vi "P116x2ch_WriteAuto.vi"(5 "P116x2":T1, 7 "Enable(T)":bool=TRUE, 8 "error in (no error)":errorcluster, 9 "RateSP":T2, 10 "NuevoSP":T2, 11 "VISA Eurotherm":refnum<visa-resource-name>) -> (0 "error out":errorcluster, 1 "RateSP_out":T2, 2 "NuevoSP_out":T2)   [LabVIEW 2017]
uses:
  2xP116.ctl
  _P2024_P116x2w.ctl
  Address.ctl
  Eurotherm_2023_Module.ctl
  P2024 TB ICB GLOBALES.vi
panel:
  out "PV":T2
  out "WorkingSP":T2
  out "TargetSP":T2
  in  "Cancel":bool
  in  "Write":bool
  in  "Delay Time (s)":dbl=0.1
  # "Setpoint auto controladores P116"
  # "C/min"
  # "C"
  # "C"
  # "C"
  # "C"
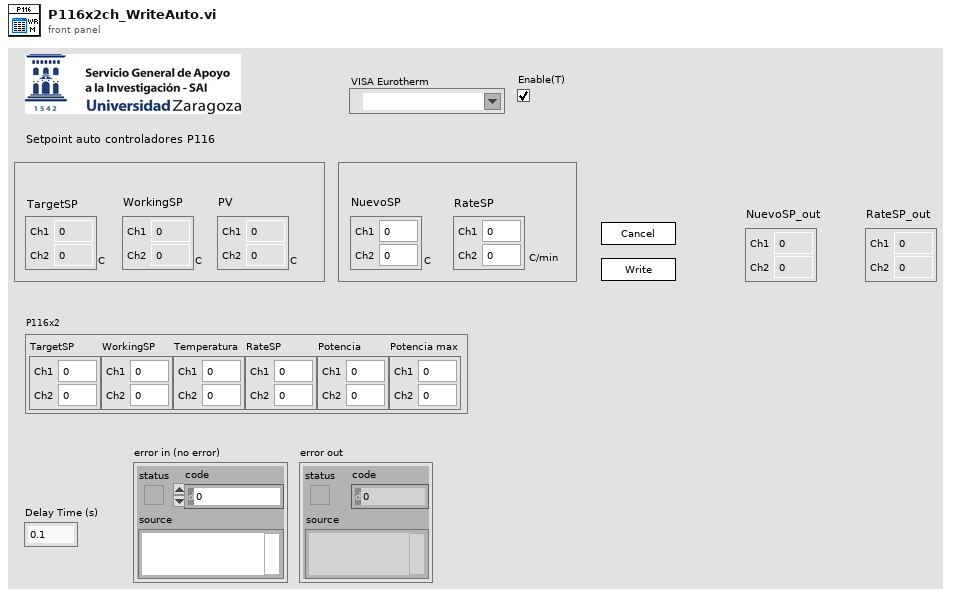
[diagram p1: front panel]
types:
  T1 = typedef "_P2024_P116x2w.ctl" = cluster{"TargetSP":T2, "WorkingSP":T2, "Temperatura":T2, "RateSP":T2, "Potencia":T2, "Potencia max":T2}
  T2 = typedef "2xP116.ctl" = cluster{"Ch1":dbl, "Ch2":dbl}
  T3 = typedef "_P2024 COMMS.ctl" = cluster{"Alicat":refnum<visa-resource-name>, "eAlic":bool, "Eurotherm":refnum<visa-resource-name>, "eEurot":bool, "Balanza":refnum<visa-resource-name>, "eBal":bool, "Valvula":refnum<visa-resource-name>, "eVal":bool}
  T4 = typedef "Eurotherm_2023_Module.ctl" = enum16{"Initialize", "Write setpoint", "Read data", "Write ramp rate", "Set constante proporcional", "Set constante integral", "Set constante diferencial", "Set ouput limit LOW", "Set ouput limit HIGH", "Shutdown"}
  T5 = typedef "Address.ctl" = enum16{"Add 1", "Add 2", "Add 3", "Add 4", "Add 5", "Add 6", "Add 10", "Add 11", "Add 12", "Add 13"}
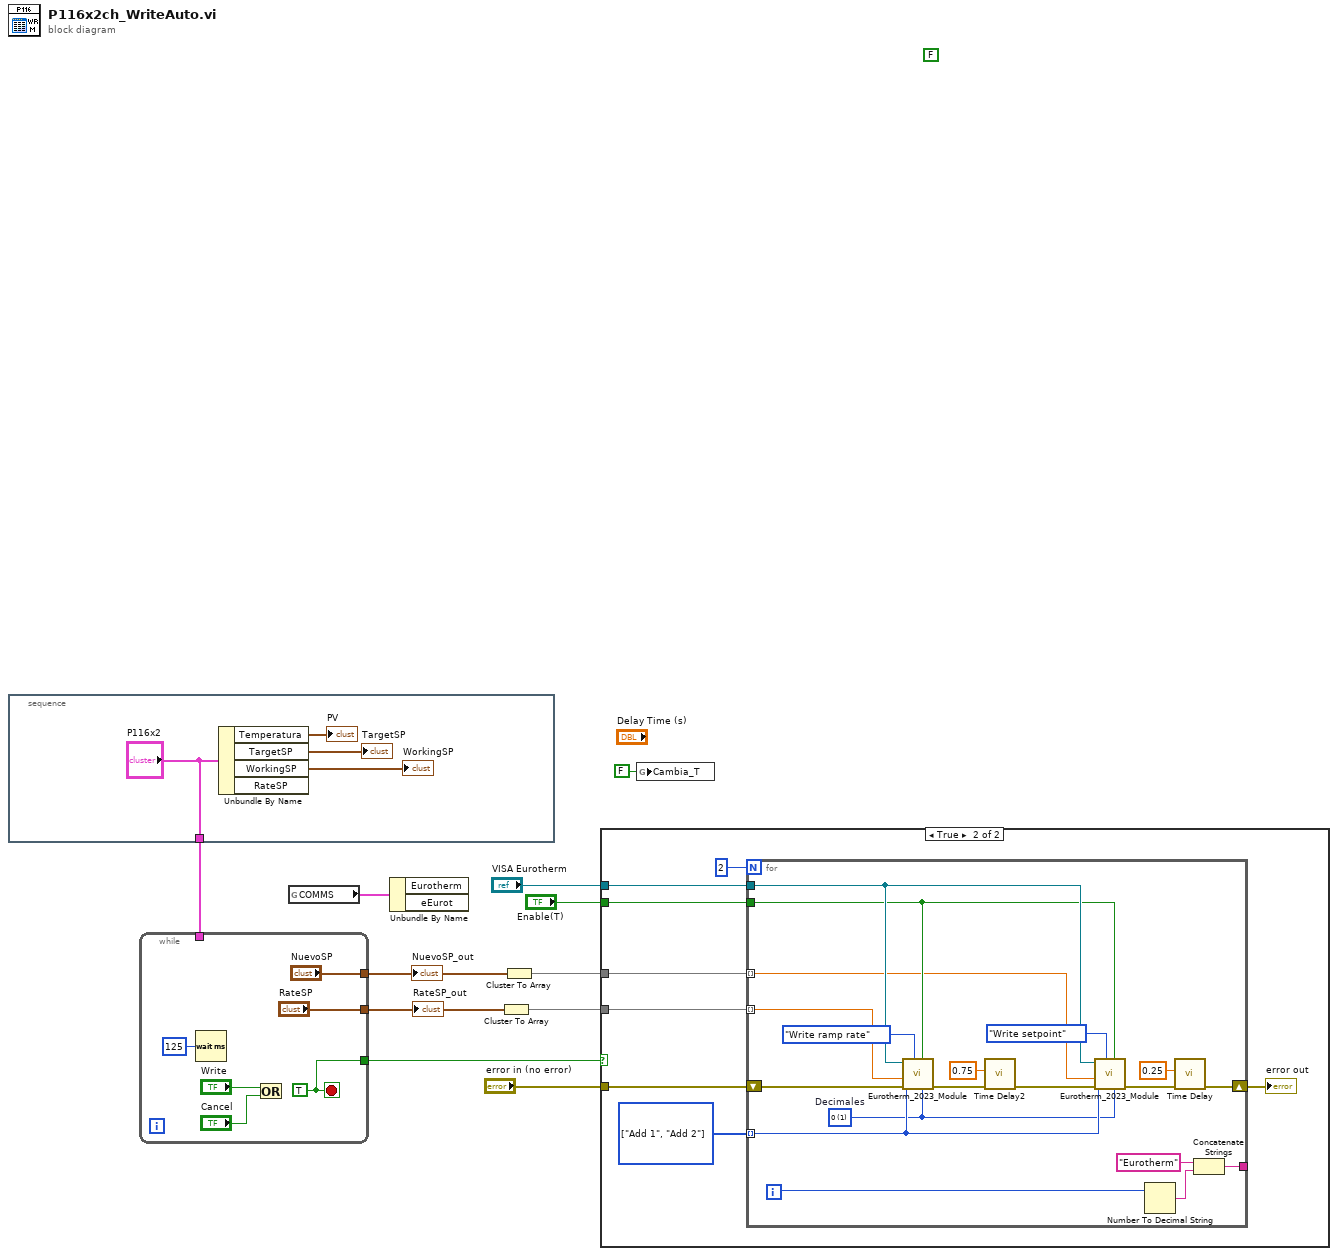
[diagram p0: block diagram]
diagram:
  (unwired) FALSE
  n1 = stacked-sequence {
    tunnel: ["P116x2"] -> w3
    frame #0 {
      n2 = Unbundle By Name("P116x2") -> ("Temperatura"=→"PV":T2, "TargetSP"=→"TargetSP":T2, "WorkingSP"=→"WorkingSP":T2)  [unwired: 1 out]
    }
  }
  n3 = while {
    tunnel: ["NuevoSP"] -> w1
    tunnel: ["RateSP"] -> w2
    tunnel: [w16] -> w6
    tunnel: w3 -> [_]
    stop <- w16 stop-if-true
    w16 = TRUE
    n4 = Wait (ms)(milliseconds to wait=u32 125) -> ()  [unwired: 1 out]
    n5 = Or(x="Write", y="Cancel") -> ()  [unwired: 1 out]
  }
  "NuevoSP_out" <- w1
  "RateSP_out" <- w2
  n6 = global read "P2024 TB ICB GLOBALES.vi" "COMMS"() -> (w11:T3)
  n7 = Unbundle By Name(w11) -> ()  [unwired: 2 out]
  n8 = Cluster To Array(cluster=w2) -> (array=w7:dbl[])
  n9 = Cluster To Array(cluster=w1) -> (array=w8:dbl[])
  n10 = case shown="True" w6 {
    tunnel: "Enable(T)" -> [_ w28]
    tunnel: "error in (no error)" -> [_ w26]
    tunnel: w8 -> [_ w24]
    tunnel: w7 -> [_ w25]
    tunnel: "VISA Eurotherm" -> [_ w29]
    frame False {
    }
    frame True {
      w22 = T5[] [enum."Add 1", enum."Add 2"] items=["Add 1", "Add 2", "Add 3", "Add 4", "Add 5", "Add 6", "Add 10", "Add 11", "Add 12", "Add 13"]
      n11 = for {
        N: 2 -> [_]
        tunnel: w22 -> [w31] mode=indexing
        shift-right: [w36] -> w27
        shift-left: w26 -> [w43]
        tunnel: [w46] -> _
        tunnel: w24 -> [w38] mode=indexing
        tunnel: w25 -> [w39] mode=indexing
        tunnel: w29 -> [w42]
        tunnel: w28 -> [w41]
        i -> [w35]
        w30 = u16 1 items=["0"=1, "1"=10, "2"=100]  # Decimales
        n12 = call "Eurotherm_2023_Module.vi"("Decimales"=w30, "Eurotherm (T:Enable)"=w41, "Command"=Eurotherm_2023_Module."Write ramp rate", "error in (no error)"=w43, "Value"=w39, "Address"=w31, "VISA resource name"=w42) -> ("error out"=w33:errorcluster)  [unwired: 3 in, 1 out]
        n13 = call "Time Delay2"("error in (no error)"=w33, "Delay Time (s)"=0.75) -> ("error out"=w32:errorcluster)  [unwired: 9 in]
        n14 = call "Eurotherm_2023_Module.vi"("Decimales"=w30, "Eurotherm (T:Enable)"=w41, "Command"=Eurotherm_2023_Module."Write setpoint", "error in (no error)"=w32, "Value"=w38, "Address"=w31, "VISA resource name"=w42) -> ("error out"=w37:errorcluster)  [unwired: 3 in, 1 out]
        n15 = Number To Decimal String(number=w35) -> (decimal integer string=w47:string)  [unwired: 1 in]
        n16 = call "Time Delay"("error in (no error)"=w37, "Delay Time (s)"=0.25) -> ("error out"=w36:errorcluster)  [unwired: 9 in]
        n17 = Concatenate Strings("Eurotherm" ("error source (\" \")"), w47) -> (w46:string)
      }
      "error out" <- w27
    }
  }
  n18 = global write "P2024 TB ICB GLOBALES.vi" "Cambia_T"(FALSE ("ChangeT")) -> ()
